vi "Untitled 14.vi"(4 "axis":u32, 5 "step":dbl, 6 "handle":i32, 7 "position":dbl, 8 "error in":errorcluster, 10 "+/-":bool, 11 "move":bool) -> (0 "error out":errorcluster)   [LabVIEW 2013]
uses:
  C:/Users/admin/Desktop/controller/SubVIs_nanostage/Madlib.dll
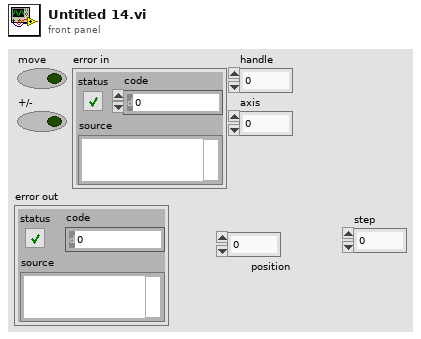
[diagram p1: front panel]
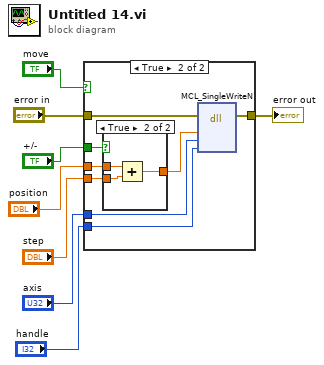
[diagram p0: block diagram]
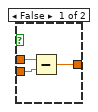
[diagram p3: hidden frame]
diagram:
  n1 = case shown="True" "move" {
    tunnel: "+/-" -> [_ w17]
    tunnel: "error in" -> [w9 w14]
    tunnel: [w9 w15] -> w3
    tunnel: "step" -> [_ w13]
    tunnel: "position" -> [_ w12]
    tunnel: "handle" -> [_ w11]
    tunnel: "axis" -> [_ w10]
    frame False {
    }
    frame True {
      n2 = case shown="True" w17 {
        tunnel: w12 -> [w19 w23]
        tunnel: [w20 w22] -> w16
        tunnel: w13 -> [w18 w21]
        frame False {
          n3 = Subtract(x=w19, y=w18) -> (x-y=w20:dbl)
        }
        frame True {
          n4 = Add(x=w23, y=w21) -> (x+y=w22:dbl)
        }
      }
      n5 = dll-call lib="C:/Users/admin/Desktop/controller/SubVIs_nanostage/MADLib.dll" fn="MCL_SingleWriteN"(error in=w14, "position"=w16, "axis"=w10, "handle"=w11) -> (error out=w15:errorcluster)  [unwired: 6 in, 1 out]
    }
  }
  "error out" <- w3
